vi "PTSequencer.constructor.vi"(0 "name":string, 2 "data in":string, 5 "error in(no error)":errorcluster) -> (14 "i ref out":refnum<vi>, 16 "data out":string, 19 "error out":errorcluster)   [LabVIEW 2014, in "PTSequencer.lvlib"]
uses:
  PTSequencer.lvlib
  CSCore/CSSystem/CoreLib/CoreLib.string 2 byte array.vi
  CSCore/CSSystem/CSSystemLib/CSSystemLib.lvlib
  CSCore/BaseProcess/BaseProcess.lvlib
  CSCore/BaseSM/BaseSM.lvlib
  CSCore/BaseGUI/BaseGUI.lvlib
  CSCore/CSObj/CSObj.lvlib
  CSCore/CSSystem/CoreLib/CoreLib.lvlib
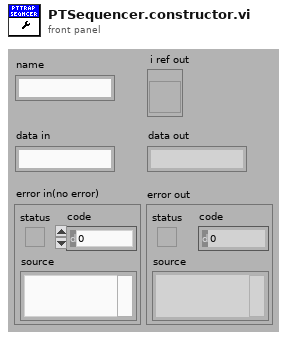
[diagram p1: front panel]
types:
  T1 = enum16{"SetAttribute", "GetAttribute", "CreateAttribute", "DestroyAttribute", "DestroyAllAtributes"}
  T2 = typedef "BaseProcess.lvlib/BaseProcess.i attribute.ctl" = cluster{"EventStatus":string, "EventError":i32, "PresetEvtWatchD":i32, "PresetPdcWatchD":i32, "EventTimeout":i32, "PeriodicInterval":i32, "Interface":string[], "Address":string[], "Special":string[], "PeriodicError":i32, "PeriodicStatus":string, "SuperProc":string, "Descriptors":T3[], "CaseRef":refnum<vi>, "PdcRef":refnum<vi>, "Thread Ref":refnum<vi>, "eventErrorID":i32, "eventStatusID":i32, "periodicErrorID":i32, "periodicStatusID":i32, "pdcCtrID":i32}
  T3 = typedef "BaseProcess.lvlib/BaseProcess.descriptor definition.ctl" = cluster{"selector":string, "descriptor":T4}
  T4 = typedef "BaseProcess.lvlib/BaseProcess.descriptor string definition.ctl" = string
  T5 = typedef "CoreDefs.rawDataType.ctl" = i8[]
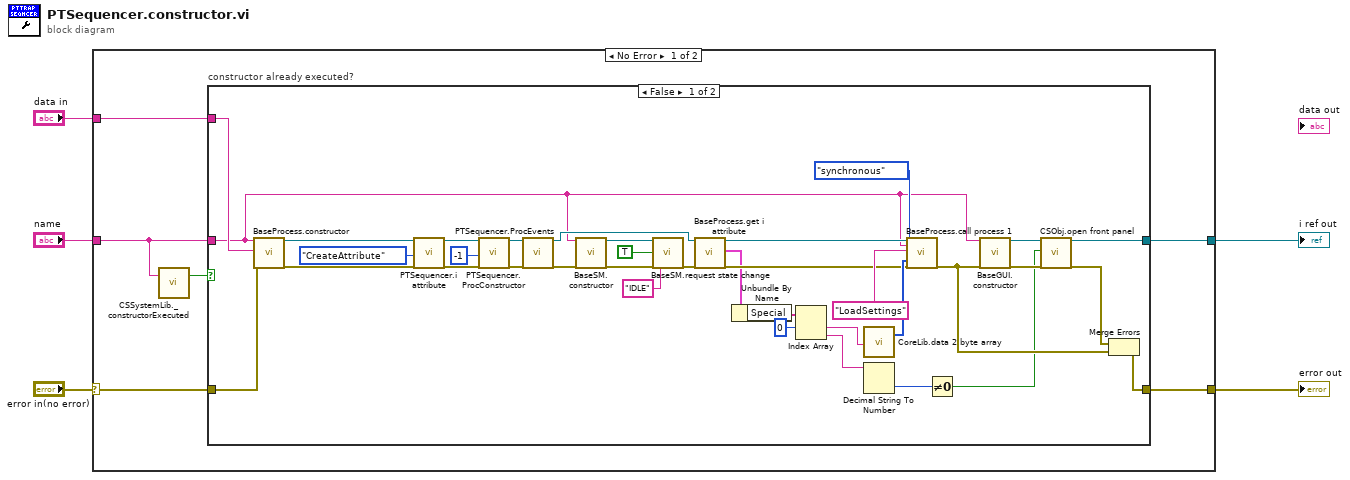
[diagram p0: block diagram]
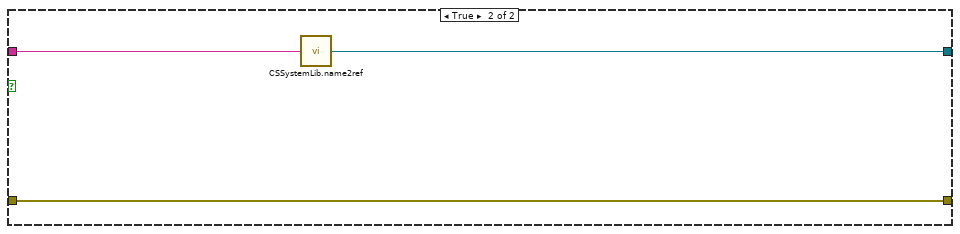
[diagram p2: hidden frame]
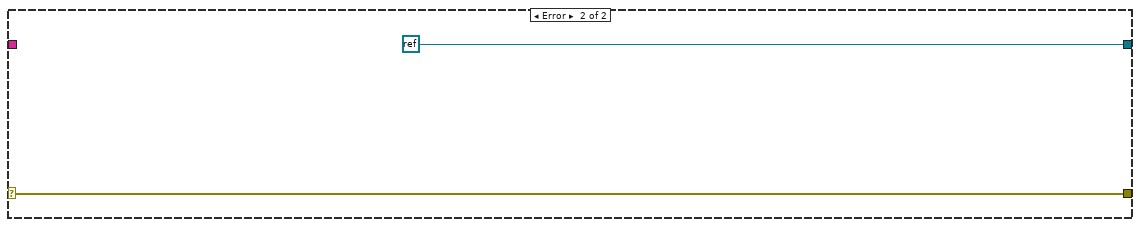
[diagram p3: hidden frame]
diagram:
  n1 = case shown="No Error" "error in(no error)" {
    selector: "error in(no error)" -> [w8 w51]
    tunnel: "name" -> [w6 _]
    tunnel: [w11 refnum<k0> refnum] -> w4
    tunnel: [w10 w51] -> w3
    tunnel: "data in" -> [w9 _]
    frame No Error {
      n2 = call "CSSystemLib._constructorExecuted.vi"("name"=w6) -> ("constructor executed?"=w7:bool)  [unwired: 18 in]
      n3 = case "constructor already executed?" shown="False" w7 {
        tunnel: w6 -> [w15 w50]
        tunnel: [w16 w49] -> w11
        tunnel: [w20 w48] -> w10
        tunnel: w9 -> [w44 _]
        tunnel: w8 -> [w43 w48]
        frame False {
          n4 = call "BaseProcess.constructor.vi"("name"=w15, "data in"=w44, "error in (no error)"=w43) -> ("i ref out"=w47:refnum<vi>, "error out"=w46:errorcluster)  [unwired: 14 in, 1 out]
          n5 = call "PTSequencer.i attribute.vi"("VI Refnum"=w47, "Action"=T1."CreateAttribute", "error in (no error)"=w46) -> ("VI Refnum out"=w37:refnum<vi>, "error out"=w34:errorcluster)  [unwired: 14 in, 1 out]
          n6 = call "PTSequencer.ProcConstructor.vi"("i ref in"=w37, "ms timeout (10000)"=-1, "error in (no error)"=w34) -> ("i ref out"=w36:refnum<vi>, "error out"=w35:errorcluster)  [unwired: 14 in, 1 out]
          n7 = call "PTSequencer.ProcEvents.vi"("i ref in"=w36, "error in"=w35) -> ("i ref out"=w29:refnum<vi>, "error out"=w38:errorcluster)  [unwired: 16 in]
          n8 = call "BaseSM.constructor.vi"("name"=w15, "error in (no error)"=w38) -> ("i ref out"=w39:refnum<vi>, "error out"=w40:errorcluster)  [unwired: 15 in, 1 out]
          n9 = call "BaseSM.request state change.vi"("i ref in"=w39, "change"=TRUE, "error in (no error)"=w40, "requested state"="IDLE") -> ("error out"=w27:errorcluster)  [unwired: 12 in, 3 out]
          n10 = call "BaseProcess.get i attribute.vi"("i ref in"=w29, "error in (no error)"=w27) -> ("i ref out"=w28:refnum<vi>, "i attribute"=w25:T2, "error out"=w26:errorcluster)  [unwired: 15 in]
          n11 = Unbundle By Name(w25) -> ("Special"=w24:string[])
          n12 = Index Array(array=w24, index #1=0 ("index")) -> (element #1=w22:string, element #2=w21:string)  [unwired: 1 in]
          n13 = call-poly "CoreLib.data 2 byte array.vi"("string"=w22) -> ("byteArray out"=w30:T5)  [unwired: 18 in]
          n14 = Decimal String To Number(string=w21) -> (number=w17:i32)  [unwired: 2 in, 1 out]
          n15 = call "BaseProcess.call process 1.vi"("i ref in"=w28, "Object"=w15, "Selector"="LoadSettings", "CallType"=enum16{"simple", "synchronous", "asynchronous"}."synchronous", "Data"=w30, "error in (no error)"=w26) -> ("error out"=w13:errorcluster)  [unwired: 11 in, 2 out]
          n16 = Not Equal To 0?(x=w17) -> (x != 0?=w12:bool)
          n17 = call "BaseGUI.constructor.vi"("name"=w15, "error in (no error)"=w13) -> ("i ref out"=w19:refnum<vi>, "error out"=w18:errorcluster)  [unwired: 15 in, 1 out]
          n18 = call "CSObj.open front panel.vi"("i ref in"=w19, "frontPanelOpen"=w12, "error in (no error)"=w18) -> ("i ref out"=w16:refnum<vi>, "error out"=w14:errorcluster)  [unwired: 15 in]
          n19 = Merge Errors(w14, w13) -> (w20:errorcluster)
        }
        frame True {
          n20 = call "CSSystemLib.name2ref.vi"("name"=w50) -> ("obj refnum"=w49:refnum<vi>)
        }
      }
    }
    frame Error {
    }
  }
  "i ref out" <- w4
  "error out" <- w3
